vi "MUX Config Const.vi"() -> (2 "MUX Config":T1[](array[typedef])=[{"Outputs"=[{"Desk Left", 2817882}, {"Desk Center", 2817882}, {"Desk Right", 2817882}, {"Bench Left", 12492800}, {"Bench Right", 12492800}, {"F", 7171459}, {"G", 7171459}, {"Mux Out", 16746514}], "Inputs"=[{"Desktop 1", 16448250}, {"Desktop 2", 16448250}, {"Desktop 3", 16448250}, {"Dock 1", 7078143}, {"Dock 2", 7078143}, {"Dock 3", 7078143}, {"Red HDMI", 16727100}, {"Mux In", 16750705}]}, {"Outputs"=[{"TV", 16775513}, {"", 0}, {"", 0}, {"", 0}, {"", 0}, {"", 0}, {"HD60S Capture", 44252}, {"Mux Out", 16750705}], "Inputs"=[{"Blu-ray", 9567230}, {"2", 0}, {"3", 0}, {"4", 0}, {"Consoles", 16711776}, {"5", 0}, {"Blue HDMI", 2768895}, {"Mux In", 16746514}]}])   [LabVIEW 2022 SP3, in "TouchControl.lvlib"]
uses:
  TouchControl.lvlib
  MUX Config.ctl
  MUX Element.ctl
  MUX Selection.ctl
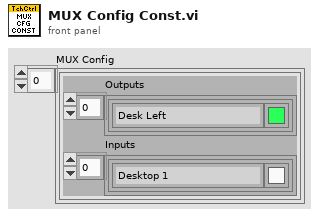
[diagram p1: front panel]
types:
  T1 = typedef "TouchControl.lvlib/MUX Config.ctl" = cluster{"Outputs":T2[], "Inputs":T2[]}
  T2 = typedef "TouchControl.lvlib/MUX Element.ctl" = cluster{string, u32}
  T3 = typedef "TouchControl.lvlib/MUX Selection.ctl" = enum16{"Computers", "Others"}
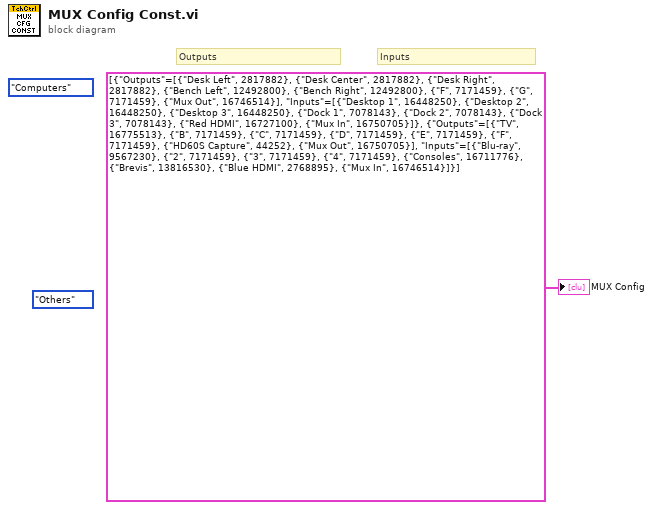
[diagram p0: block diagram]
diagram:
  (unwired) MUX_Selection."Others" ("MUX Selection")
  (unwired) MUX_Selection."Computers" ("MUX Selection")
  # "Inputs"
  # "Outputs"
  "MUX Config" <- T1[] [{"Outputs"=[{"Desk Left", 2817882}, {"Desk Center", 2817882}, {"Desk Right", 2817882}, {"Bench Left", 12492800}, {"Bench Right", 12492800}, {"F", 7171459}, {"G", 7171459}, {"Mux Out", 16746514}], "Inputs"=[{"Desktop 1", 16448250}, {"Desktop 2", 16448250}, {"Desktop 3", 16448250}, {"Dock 1", 7078143}, {"Dock 2", 7078143}, {"Dock 3", 7078143}, {"Red HDMI", 16727100}, {"Mux In", 16750705}]}, {"Outputs"=[{"TV", 16775513}, {"B", 7171459}, {"C", 7171459}, {"D", 7171459}, {"E", 7171459}, {"F", 7171459}, {"HD60S Capture", 44252}, {"Mux Out", 16750705}], "Inputs"=[{"Blu-ray", 9567230}, {"2", 7171459}, {"3", 7171459}, {"4", 7171459}, {"Consoles", 16711776}, {"Brevis", 13816530}, {"Blue HDMI", 2768895}, {"Mux In", 16746514}]}]
